vi "Operator Panel 2D_v2.vi"() -> ()   [LabVIEW 2009]
doc: "This VI is an example operator panel.\n\nThe VI contains a table for the field values that may be configured manually, or loaded by checking the \"Prompt for File\" box. The data file should contain 3 columns of data, with each column delimited by a tab character.\n\nBefore the VI is executed, set the desired field units and coordinate system. Once the VI is started, follow the directions in the STATUS indicator to operate. Once a field value is achieved, it will be held indefinitely with no user intervention.\n\nThe present field is displayed in the selected units and coordinate system. The present field is queried once per second.\n\nIf a field point is specified that is outside the limits for the magnet, the VI will abort execution."
uses:
  <vilib>/Utility/file.llb/Read From Spreadsheet File (DBL).vi
panel:
  in  "Z-Axis Communications Config":T1={"GPIB address"=22, "GPIB bus"=1, "connection ID"=refnum, "IP"="192.168.20.40", "Active Comm Interface"=0, "Serial Port"="", "Programmer Type"=0} {"Programmer Type" items=["Model 430", "Model 420"]; "Active Comm Interface" items=["TCP/IP (Model 430 Only)", "RS232", "IEEE488"]}
  in  "Max Ramp Rate - Y Axis (A/s)":dbl=0.065 format="%.3f"
  in  "Max Ramp Rate - Z Axis (A/s)":dbl=0.203 format="%.3f"
  in  "Magnitude Limit (kG)":dbl=45.1 format="%.3f"
  in  "Y-Axis Communications Config":T1={"GPIB address"=22, "GPIB bus"=1, "connection ID"=refnum, "IP"="192.168.20.32", "Active Comm Interface"=0, "Serial Port"="", "Programmer Type"=0} {"Programmer Type" items=["Model 430", "Model 420"]; "Active Comm Interface" items=["TCP/IP (Model 430 Only)", "RS232", "IEEE488"]}
  out "Cartesian Display (T)":T2 {"Z-Axis Field (T)" format="%.3f"; "Y-Axis Field (T)" format="%.3f"}
  in  "Starting index":i32 min=0 max=17 step=1
  in  "Normal color":u32(colorbox)=11711154
  in  "Highlight color":u32(colorbox)=16711680
  out "?":string="American Magnetics, Inc."
  in  "Prompt for File?":bool
  out "Continue Execution?":bool=TRUE
  out "error out":T3
  in  "error in":T3
  out "STATUS":string
  in  "Ramping Control":u16(ring)=3 items=["NEXT VECTOR", "RAMPING", "HOLDING", "PAUSE", "ZERO"]
  out "Cartesian Display (kG)":T4 {"Z-Axis Field (kG)" format="%.3f"; "Y-Axis Field (kG)" format="%.3f"}
  in  "Field Values":string[][](table)
  out "Switch Heaters":bool
  out "Polar Display (T)":T5 {"Z-Axis Field (T)" format="%.3f"; "q (degrees)" format="%.3f"}
  out "Polar Display (kG)":T6 {"Z-Axis Field (kG)" format="%.3f"; "q (degrees)" format="%.3f"}
  in  "Coordinate System":u16(ring) items=["Cartesian", "Polar"]
  in  "Magnetic Field Units":u16(ring) items=["kG", "Tesla"]
  # "Configuration and Status"
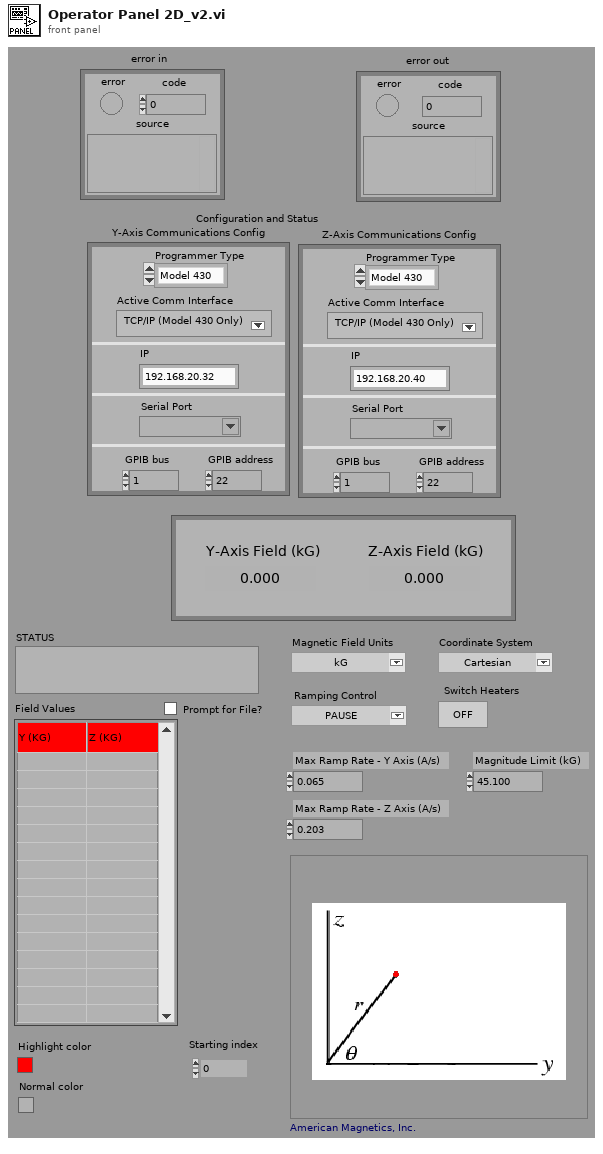
[diagram p1: front panel]
types:
  T1 = cluster{"GPIB address":i16, "GPIB bus":i16, "connection ID":refnum<k5>, "IP":string, "Active Comm Interface":u16, "Serial Port":refnum<visa-resource-name>, "Programmer Type":u16}
  T2 = cluster{"Y-Axis Field (T)":dbl, "Z-Axis Field (T)":dbl}
  T3 = cluster{"error":bool, "code":i32, "source":string}
  T4 = cluster{"Y-Axis Field (kG)":dbl, "Z-Axis Field (kG)":dbl}
  T5 = cluster{"q (degrees)":dbl, "Z-Axis Field (T)":dbl}
  T6 = cluster{"q (degrees)":dbl, "Z-Axis Field (kG)":dbl}
  T7 = enum16{"", "RAMPING", "HOLDING", "PAUSED", "MANUAL UP", "MANUAL DOWN", "ZEROING CURRENT", "QUENCH DETECTED", "HEATING SWITCH"}
  T8 = enum16{"", "RAMPING", "HOLDING", "PAUSED", "MANUAL UP", "MANUAL DOWN", "ZEROING CURRENT", "QUENCH DETECTED", "HEATING SWITCH", "AT ZER0", "COOLING SWITCH"}
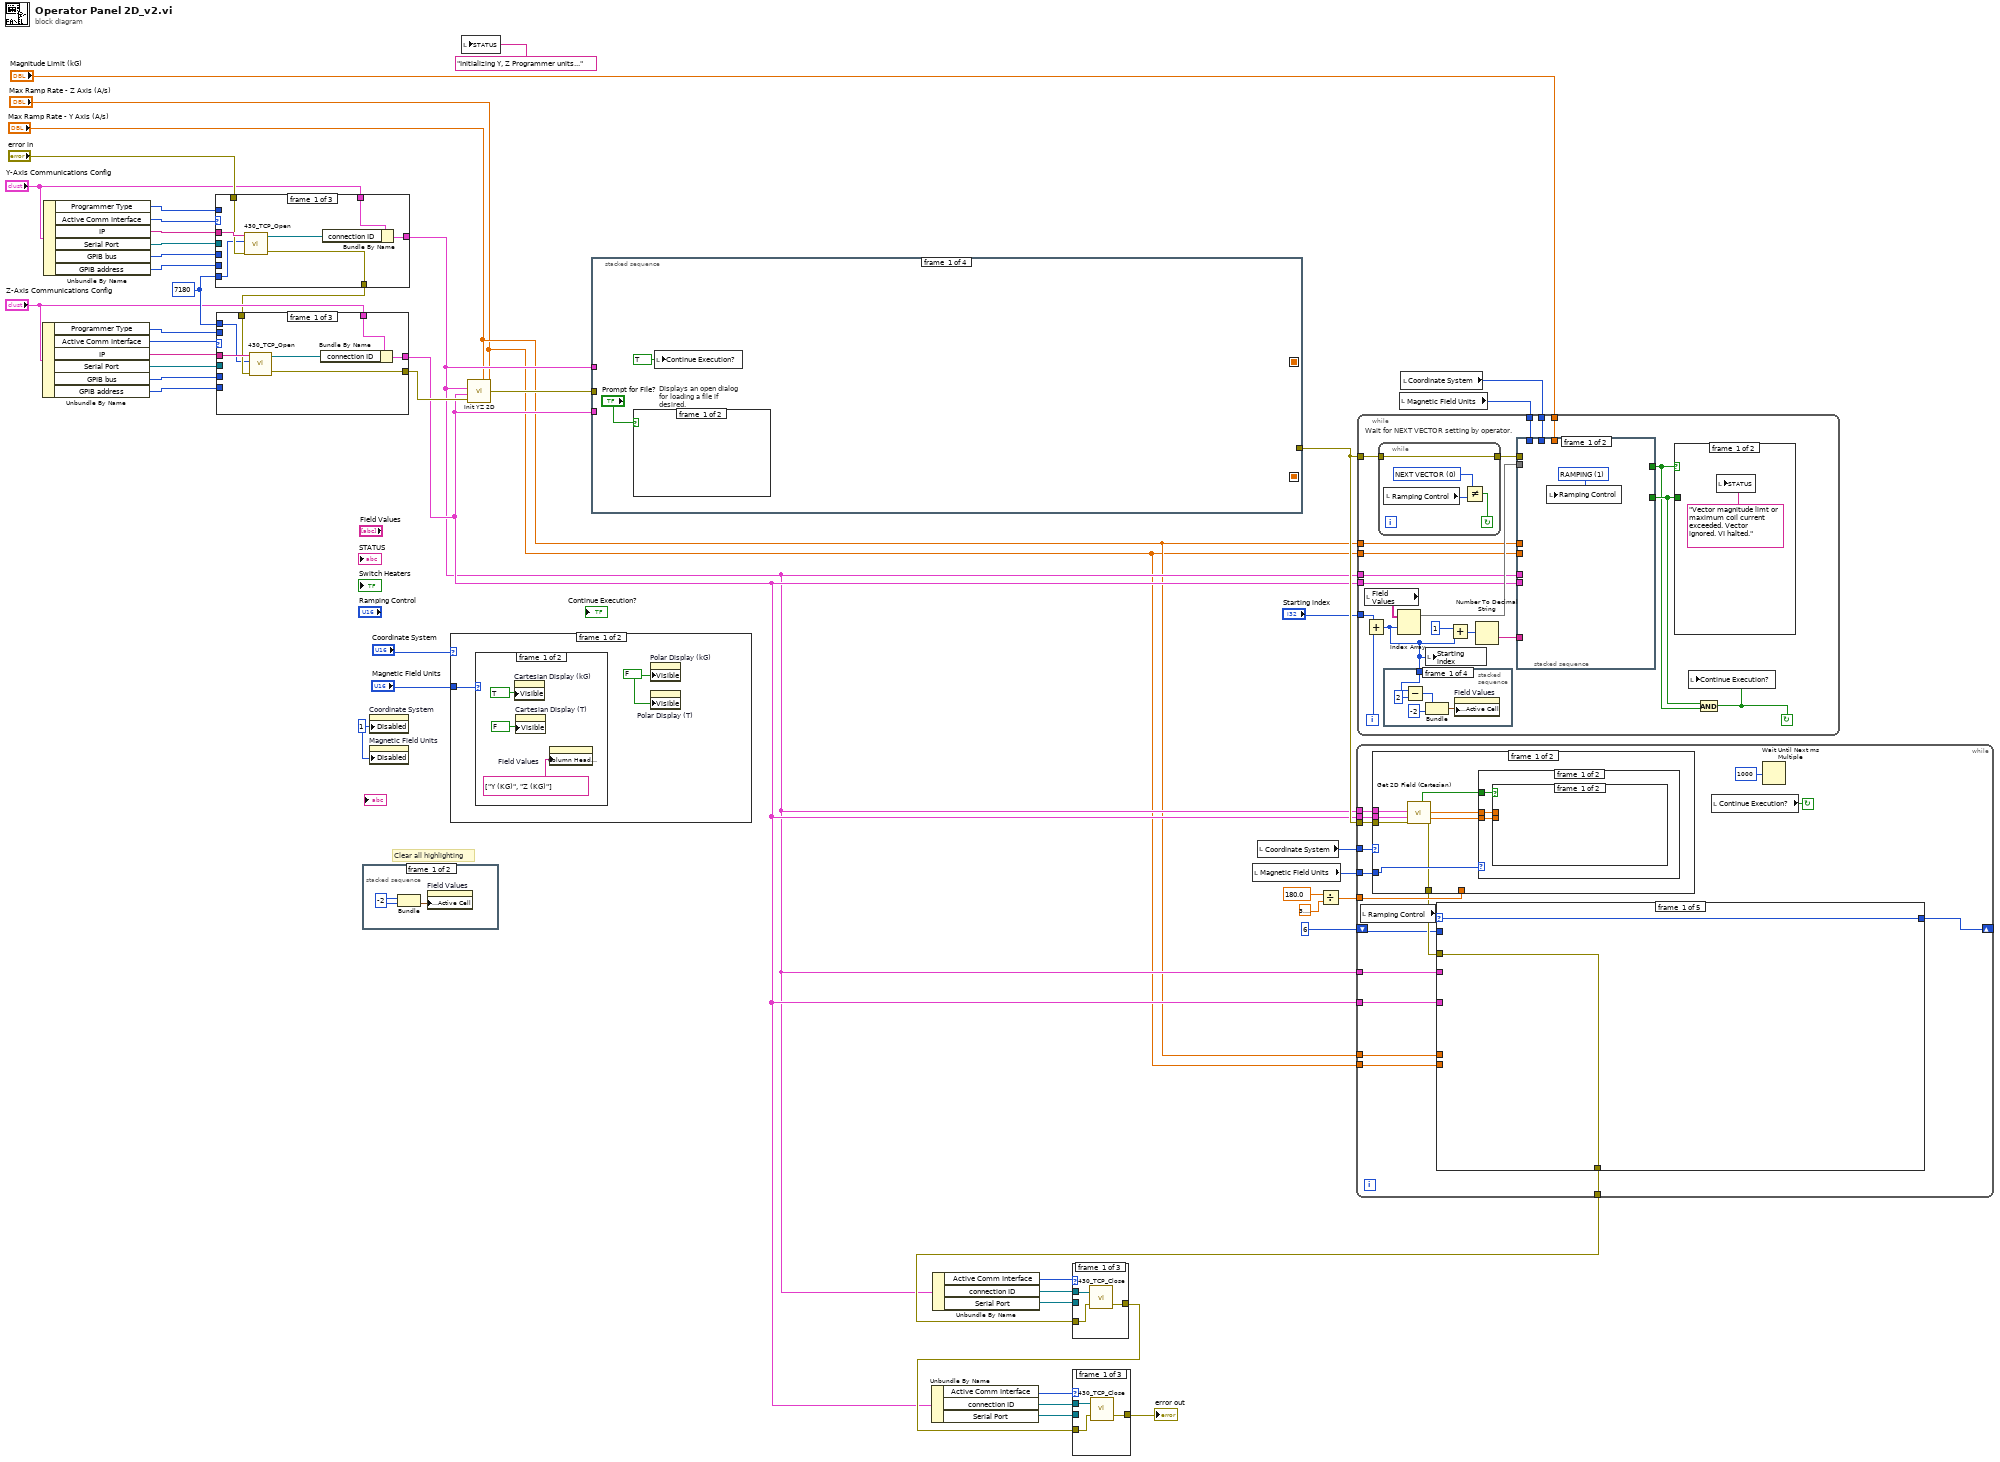
[diagram p0: block diagram]
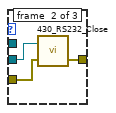
[diagram p2: hidden frame]
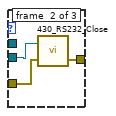
[diagram p4: hidden frame]
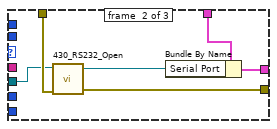
[diagram p6: hidden frame]
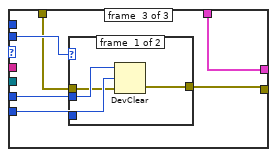
[diagram p7: hidden frame]
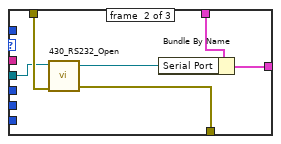
[diagram p9: hidden frame]
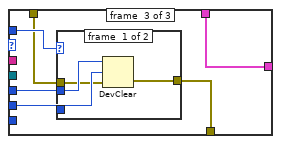
[diagram p10: hidden frame]
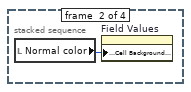
[diagram p12: hidden frame]
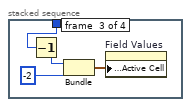
[diagram p13: hidden frame]
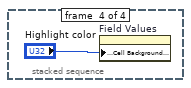
[diagram p14: hidden frame]
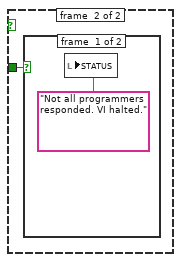
[diagram p15: hidden frame]
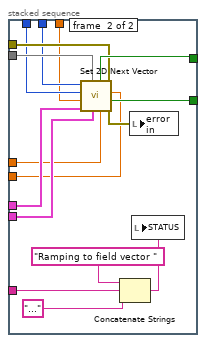
[diagram p17: hidden frame]
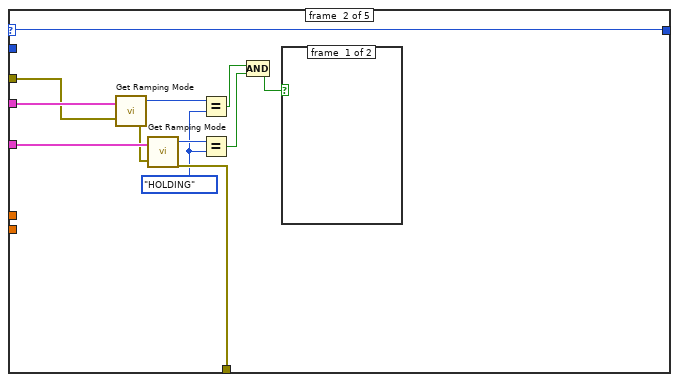
[diagram p18: hidden frame]
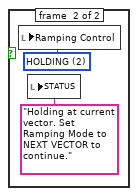
[diagram p19: hidden frame]
diagram:
  w32 = 7180 ("TCP Port")
  w45 = u8 1 ("Write Attribute")
  # "Clear all highlighting"
  n1 = Unbundle By Name("Z-Axis Communications Config") -> ("Programmer Type"=w7:u16, "Active Comm Interface"=w31:u16, "IP"=w28:string, "Serial Port"=w27:refnum<visa-resource-name>, "GPIB bus"=w6:i16, "GPIB address"=w5:i16)
  n2 = Unbundle By Name("Y-Axis Communications Config") -> ("Programmer Type"=w1:u16, "Active Comm Interface"=w30:u16, "IP"=w29:string, "Serial Port"=w26:refnum<visa-resource-name>, "GPIB bus"=w2:i16, "GPIB address"=w3:i16)
  n3 = case shown="2" w30 {
    tunnel: w29 -> [w54 _ _]
    tunnel: "error in" -> [w53 w60 w62]
    tunnel: "Y-Axis Communications Config" -> [w52 w55 w66]
    tunnel: [w50 w58 w66] -> w14
    tunnel: [w49 w59 w61] -> w4
    tunnel: w32 -> [w48 _ _]
    tunnel: w26 -> [_ w56 _]
    tunnel: w3 -> [_ _ w65]
    tunnel: w2 -> [_ _ w64]
    tunnel: w1 -> [_ _ w63]
    frame #0 {
      n4 = call <userlib>:"430_TCP_Open.vi"("IP Address"=w54, "TCP Port"=w48, "error in (no error)"=w53) -> ("connection ID"=w51:refnum<k5>, "error out"=w49:errorcluster)  [unwired: 3 in, 1 out]
      n5 = Bundle By Name(cluster=w52, "connection ID"=w51) -> (w50:T1)
    }
    frame #1 {
      n6 = call <userlib>:"430_RS232_Open.vi"("VISA resource name"=w56, "error in (no error)"=w60) -> ("VISA resource name out"=w57:refnum<visa-resource-name>, "error out"=w59:errorcluster)  [unwired: 5 in]
      n7 = Bundle By Name(cluster=w55, "Serial Port"=w57) -> (w58:T1)
    }
    frame #2 {
      n8 = case shown="0, Default" w63 {
        tunnel: w64 -> [w70 _]
        tunnel: w65 -> [w69 _]
        tunnel: w62 -> [w68 w71]
        tunnel: [w67 w71] -> w61
        frame #0 {
          n9 = DevClear(2:w68, 3:w69, 4:w70) -> (0:w67:errorcluster)  [unwired: 1 out]
        }
        frame #1 {
        }
      }
    }
  }
  n10 = case shown="2" w31 {
    tunnel: w28 -> [w78 _ _]
    tunnel: w4 -> [w77 w84 w86]
    tunnel: [w76 w83 w85] -> w24
    tunnel: "Z-Axis Communications Config" -> [w75 w81 w90]
    tunnel: [w73 w82 w90] -> w15
    tunnel: w32 -> [w72 _ _]
    tunnel: w27 -> [_ w79 _]
    tunnel: w7 -> [_ _ w89]
    tunnel: w6 -> [_ _ w88]
    tunnel: w5 -> [_ _ w87]
    frame #0 {
      n11 = call <userlib>:"430_TCP_Open.vi"("IP Address"=w78, "TCP Port"=w72, "error in (no error)"=w77) -> ("connection ID"=w74:refnum<k5>, "error out"=w76:errorcluster)  [unwired: 3 in, 1 out]
      n12 = Bundle By Name(cluster=w75, "connection ID"=w74) -> (w73:T1)
    }
    frame #1 {
      n13 = call <userlib>:"430_RS232_Open.vi"("VISA resource name"=w79, "error in (no error)"=w84) -> ("VISA resource name out"=w80:refnum<visa-resource-name>, "error out"=w83:errorcluster)  [unwired: 5 in]
      n14 = Bundle By Name(cluster=w81, "Serial Port"=w80) -> (w82:T1)
    }
    frame #2 {
      n15 = case shown="0, Default" w89 {
        tunnel: w88 -> [w94 _]
        tunnel: w87 -> [w93 _]
        tunnel: w86 -> [w92 w95]
        tunnel: [w91 w95] -> w85
        frame #0 {
          n16 = DevClear(2:w92, 3:w93, 4:w94) -> (0:w91:errorcluster)  [unwired: 1 out]
        }
        frame #1 {
        }
      }
    }
  }
  n17 = stacked-sequence {
    frame #0 {
      w96 = -2
      n18 = Bundle(w96, w96) -> (w97:cluster{i32, i32})  [unwired: 1 in]
      n19 = property on="Field Values" class="Tbl (strict)"("Active Cell:Active Cell"=w97) -> ()  [unwired: 2 in, 2 out]
    }
    frame #1 {
      n20 = property on="Field Values" class="Tbl (strict)"("Active Cell:Cell Background Color"="Normal color") -> ()  [unwired: 2 in, 2 out]
    }
  }
  n21 = property on="Coordinate System" class="Ring (strict)"("Disabled"=w45) -> ()  [unwired: 2 in, 2 out]
  n22 = property on="Magnetic Field Units" class="Ring (strict)"("Disabled"=w45) -> ()  [unwired: 2 in, 2 out]
  n23 = case shown="0, Default" "Coordinate System" {
    tunnel: "Magnetic Field Units" -> [w100 w108]
    frame #0 {
      w99 = FALSE ("Write Attribute")
      (unwired) FALSE ("Write Attribute")
      (unwired) TRUE ("Write Attribute")
      n24 = case shown="1" w100 {
        frame #0 {
          n25 = property on="Cartesian Display (kG)" class="Cluster (strict)"("Visible"=TRUE ("Write Attribute")) -> ()  [unwired: 2 in, 2 out]
          n26 = property on="Cartesian Display (T)" class="Cluster (strict)"("Visible"=FALSE ("Write Attribute")) -> ()  [unwired: 2 in, 2 out]
          n27 = property on="Field Values" class="Tbl (strict)"("Column Header Strings[]"=string[] ["Y (KG)", "Z (KG)"] ("Write Attribute")) -> ()  [unwired: 2 in, 2 out]
        }
        frame #1 {
          n28 = property on="Cartesian Display (kG)" class="Cluster (strict)"("Visible"=FALSE ("Write Attribute")) -> ()  [unwired: 2 in, 2 out]
          n29 = property on="Cartesian Display (T)" class="Cluster (strict)"("Visible"=TRUE ("Write Attribute")) -> ()  [unwired: 2 in, 2 out]
          n30 = property on="Field Values" class="Tbl (strict)"("Column Header Strings[]"=string[] ["Y (T)", "Z (T)"] ("Write Attribute")) -> ()  [unwired: 2 in, 2 out]
        }
      }
      n31 = property on="Polar Display (kG)" class="Cluster (strict)"("Visible"=w99) -> ()  [unwired: 2 in, 2 out]
      n32 = property on="Polar Display (T)" class="Cluster (strict)"("Visible"=w99) -> ()  [unwired: 2 in, 2 out]
    }
    frame #1 {
      (unwired) FALSE ("Write Attribute")
      (unwired) TRUE ("Write Attribute")
      w107 = FALSE ("Write Attribute")
      n33 = case shown="0, Default" w108 {
        frame #0 {
          n34 = property on="Polar Display (kG)" class="Cluster (strict)"("Visible"=TRUE ("Write Attribute")) -> ()  [unwired: 2 in, 2 out]
          n35 = property on="Polar Display (T)" class="Cluster (strict)"("Visible"=FALSE ("Write Attribute")) -> ()  [unwired: 2 in, 2 out]
          n36 = property on="Field Values" class="Tbl (strict)"("Column Header Strings[]"=string[] ["Mag. r (KG)", "Theta (deg)"] ("Write Attribute")) -> ()  [unwired: 2 in, 2 out]
        }
        frame #1 {
          n37 = property on="Polar Display (kG)" class="Cluster (strict)"("Visible"=FALSE ("Write Attribute")) -> ()  [unwired: 2 in, 2 out]
          n38 = property on="Polar Display (T)" class="Cluster (strict)"("Visible"=TRUE ("Write Attribute")) -> ()  [unwired: 2 in, 2 out]
          n39 = property on="Field Values" class="Tbl (strict)"("Column Header Strings[]"=string[] ["Mag. r (T)", "Theta (deg)"] ("Write Attribute")) -> ()  [unwired: 2 in, 2 out]
        }
      }
      n40 = property on="Cartesian Display (kG)" class="Cluster (strict)"("Visible"=w107) -> ()  [unwired: 2 in, 2 out]
      n41 = property on="Cartesian Display (T)" class="Cluster (strict)"("Visible"=w107) -> ()  [unwired: 2 in, 2 out]
    }
  }
  n42 = local write "STATUS"("Initializing Y, Z Programmer units..." ("STATUS")) -> ()
  n43 = call <userlib>:"Init YZ 2D.vi"("Max Ramp Rate Z-axis"="Max Ramp Rate - Z Axis (A/s)", "Max Ramp Rate Y-axis"="Max Ramp Rate - Y Axis (A/s)", "error in"=w24, "Z-Axis Communications Config"=w15, "Y-Axis Communications Config"=w14) -> ("error out"=w43:T3)  [unwired: 5 in]
  n44 = stacked-sequence {
    seq-local: [_ w122 _ _] -> [_ _ w169 _]
    seq-local: [_ w121 _ _] -> [_ _ w168 _]
    tunnel: w15 -> [_ w124 _ _]
    tunnel: w43 -> [_ w125 _ _]
    tunnel: [_ w120 _ _] -> w39
    tunnel: w14 -> [_ w123 _ _]
    frame #0 {
      n45 = case "Displays an open dialog for loading a file if desired." shown="True" "Prompt for File?" {
        frame #0 {
        }
        frame #1 {
          n46 = call-poly <vilib>:"Read From Spreadsheet File.vi"() -> ("all rows"=w119:dbl[][])  [unwired: 7 in, 4 out]
          n47 = Number To Fractional String(number=w119, precision (6)=i16 4) -> (F-format string=w118:string[][])  [unwired: 2 in]
          n48 = local write "Field Values"(w118) -> ()
        }
      }
      n49 = local write "Continue Execution?"(TRUE ("Continue Execution?")) -> ()
    }
    frame #1 {
      w133 = u16 3 items=["NEXT VECTOR", "RAMPING", "HOLDING", "PAUSE", "ZERO"] ("Ramping Control")
      n50 = call <userlib>:"Get Switch Present.vi"("error in"=w125, "Communications Config"=w123) -> ("error out"=w129:T3, "Switch Present?"=w130:bool)
      n51 = case shown="True" w130 {
        tunnel: w129 -> [w151 w160]
        tunnel: w123 -> [_ w153]
        tunnel: [0.0 w157] -> w121
        tunnel: [w151 w159] -> w128
        frame #0 {
        }
        frame #1 {
          n52 = call <userlib>:"Get Switch Heater Time.vi"("error in"=w160, "Communications Config"=w153) -> ("error out"=w156:T3, "Switch Heating Time (secs)"=w158:dbl)
          n53 = call <userlib>:"Get Switch Heater.vi"("error in"=w156, "Communications Config"=w153) -> ("error out"=w155:T3, "Switch Heater Indicator"=w154:bool)
          n54 = case shown="False" w154 {
            tunnel: [w165 w166] -> w159
            tunnel: w158 -> [w163 _]
            tunnel: [w163 0.0] -> w157
            tunnel: w155 -> [w161 w166]
            tunnel: w153 -> [w162 _]
            frame #0 {
              n55 = call <userlib>:"Set Switch Heater.vi"("error in"=w161, "Switch Heater Control"=TRUE, "Communications Config"=w162) -> ("error out"=w165:T3)
            }
            frame #1 {
            }
          }
        }
      }
      n56 = call <userlib>:"Get Switch Present.vi"("error in"=w128, "Communications Config"=w124) -> ("error out"=w126:T3, "Switch Present?"=w127:bool)
      n57 = case shown="True" w127 {
        tunnel: w126 -> [w134 w143]
        tunnel: w124 -> [_ w136]
        tunnel: [0.0 w140] -> w122
        tunnel: [w134 w142] -> w120
        frame #0 {
        }
        frame #1 {
          n58 = call <userlib>:"Get Switch Heater Time.vi"("error in"=w143, "Communications Config"=w136) -> ("error out"=w139:T3, "Switch Heating Time (secs)"=w141:dbl)
          n59 = call <userlib>:"Get Switch Heater.vi"("error in"=w139, "Communications Config"=w136) -> ("error out"=w138:T3, "Switch Heater Indicator"=w137:bool)
          n60 = case shown="False" w137 {
            tunnel: [w144 w149] -> w142
            tunnel: w141 -> [w147 _]
            tunnel: [w147 0.0] -> w140
            tunnel: w138 -> [w145 w149]
            tunnel: w136 -> [w146 _]
            frame #0 {
              n61 = call <userlib>:"Set Switch Heater.vi"("error in"=w145, "Switch Heater Control"=TRUE, "Communications Config"=w146) -> ("error out"=w144:T3)
            }
            frame #1 {
            }
          }
        }
      }
      n62 = local write "Ramping Control"(w133) -> ()
      n63 = local write "Switch Heaters"(TRUE ("Switch Heater Control")) -> ()
      n64 = property on="Switch Heaters" class="Boolean (strict)"("Disabled"=u8 1 ("Write Attribute")) -> ()  [unwired: 2 in, 2 out]
    }
    frame #2 {
      n65 = Max & Min(x=w169, y=w168) -> (max(x,y)=w170:dbl)  [unwired: 1 out]
      n66 = local write "STATUS"("Heating switches..." ("STATUS")) -> ()
      n67 = Add(x=w170, y=2) -> (x+y=w174:dbl)
      n68 = property on="Ramping Control" class="Ring (strict)"("Disabled"=u8 1 ("Write Attribute")) -> ()  [unwired: 2 in, 2 out]
      n69 = Multiply(x=w174, y=1000) -> (x*y=w173:dbl)
      n70 = Wait (ms)(milliseconds to wait=w173) -> ()  [unwired: 1 out]
    }
    frame #3 {
      n71 = property on="Ramping Control" class="Ring (strict)"("Disabled"=u8 0 ("Write Attribute")) -> ()  [unwired: 2 in, 2 out]
      n72 = local write "STATUS"("Ready to ramp to first vector. Set Ramping Mode to NEXT VECTOR to begin." ("STATUS")) -> ()
    }
  }
  n73 = Unbundle By Name(w15) -> ("Active Comm Interface"=w21:u16, "connection ID"=w20:refnum<k5>, "Serial Port"=w19:refnum<visa-resource-name>)
  n74 = Unbundle By Name(w14) -> ("Active Comm Interface"=w22:u16, "connection ID"=w18:refnum<k5>, "Serial Port"=w17:refnum<visa-resource-name>)
  n75 = local read "Magnetic Field Units"() -> (w38:u16)
  n76 = local read "Coordinate System"() -> (w40:u16)
  n77 = Divide(x=180.0, y=3.141592653589793) -> (x/y=w35:dbl)
  n78 = while {
    shift-left: u16 6 ("Ramping Control") -> [w181]
    shift-right: [w182] -> _
    tunnel: [w184] -> w16
    tunnel: w15 -> [w186]
    tunnel: w14 -> [w187]
    tunnel: w35 -> [w189]
    tunnel: w38 -> [w190]
    tunnel: w39 -> [w191]
    tunnel: w15 -> [w192]
    tunnel: w14 -> [w193]
    tunnel: w40 -> [w194]
    tunnel: "Max Ramp Rate - Y Axis (A/s)" -> [w180]
    tunnel: "Max Ramp Rate - Z Axis (A/s)" -> [w179]
    stop <- w183 continue-if-true
    n79 = local read "Ramping Control"() -> (w188:u16)
    n80 = case shown="0, Default" w194 {
      tunnel: w193 -> [w257 w281]
      tunnel: w192 -> [w256 w280]
      tunnel: w191 -> [w255 w279]
      tunnel: w190 -> [w254 w278]
      tunnel: w189 -> [_ w275]
      tunnel: [w250 w273] -> w185
      frame #0 {
        n81 = call <userlib>:"Get 2D Field (Cartesian).vi"("Y-Axis Communications Config"=w257, "Z-Axis Communications Config"=w256, "error in"=w255) -> ("All Instruments Responded?"=w251:bool, "Y-Axis Field (kG)"=w253:dbl, "Z-Axis Field (kG)"=w252:dbl, "error out"=w250:T3)  [unwired: 2 in]
        n82 = case shown="0, Default" w254 {
          tunnel: w253 -> [w260 w266]
          tunnel: w252 -> [w259 w267]
          tunnel: w251 -> [w258 w269]
          frame #0 {
            n83 = case shown="True" w258 {
              tunnel: w260 -> [_ w262]
              tunnel: w259 -> [_ w261]
              frame #0 {
              }
              frame #1 {
                n84 = Bundle("Y-Axis Field (kG)"=w262, "Z-Axis Field (kG)"=w261) -> (→"Cartesian Display (kG)":T4)  [unwired: 1 in]
              }
            }
          }
          frame #1 {
            w268 = 0.1 ("y")
            n85 = Multiply(x=w266, y=w268) -> (x*y=w265:dbl)
            n86 = Multiply(x=w267, y=w268) -> (x*y=w264:dbl)
            n87 = case shown="True" w269 {
              tunnel: w265 -> [_ w272]
              tunnel: w264 -> [_ w271]
              frame #0 {
              }
              frame #1 {
                n88 = Bundle(w272, w271) -> (→"Cartesian Display (T)":cluster{dbl, dbl})  [unwired: 1 in]
              }
            }
          }
        }
      }
      frame #1 {
        n89 = call <userlib>:"Get 2D Field (Polar).vi"("Y-Axis Communications Config"=w281, "Z-Axis Communications Config"=w280, "error in"=w279) -> ("All Instruments Responded?"=w274:bool, "Radial (r) Field (kG)"=w277:dbl, "q (radians)"=w276:dbl, "error out"=w273:T3)  [unwired: 2 in]
        n90 = case shown="0, Default" w278 {
          tunnel: w277 -> [w286 w295]
          tunnel: w276 -> [w284 w294]
          tunnel: w275 -> [w283 w293]
          tunnel: w274 -> [w285 w292]
          frame #0 {
            n91 = Multiply(x=w284, y=w283) -> (x*y=w282:dbl)
            n92 = case shown="True" w285 {
              tunnel: w286 -> [_ w289]
              tunnel: w282 -> [_ w288]
              frame #0 {
              }
              frame #1 {
                n93 = Bundle("Radial (r) Field (kG)"=w289, w288) -> (→"Polar Display (kG)":cluster{"Radial (r) Field (kG)":dbl, dbl})  [unwired: 1 in]
              }
            }
          }
          frame #1 {
            n94 = Multiply(x=w295, y=0.1) -> (x*y=w291:dbl)
            n95 = Multiply(x=w294, y=w293) -> (x*y=w290:dbl)
            n96 = case shown="True" w292 {
              tunnel: w291 -> [_ w299]
              tunnel: w290 -> [_ w298]
              frame #0 {
              }
              frame #1 {
                n97 = Bundle(w299, w298) -> (→"Polar Display (T)":cluster{dbl, dbl})  [unwired: 1 in]
              }
            }
          }
        }
      }
    }
    n98 = case shown="3" w188 {
      selector: w188 -> [w196 w206 w213 w216 w231]
      tunnel: w187 -> [_ w209 _ w220 w237]
      tunnel: w186 -> [_ w208 _ w219 w236]
      tunnel: w185 -> [w197 w201 w212 w218 w235]
      tunnel: [w197 w207 w212 w217 w234] -> w184
      tunnel: [w196 w206 w213 w216 w231] -> w182
      tunnel: w181 -> [_ _ _ w215 w233]
      tunnel: w180 -> [_ _ _ _ w230]
      tunnel: w179 -> [_ _ _ _ w229]
      frame #0 {
      }
      frame #1 {
        w200 = T7."HOLDING" ("y")
        n99 = call <userlib>:"Get Ramping Mode.vi"("Communications Config"=w209, "error in"=w201) -> ("Ramping Mode"=w204:T8, "error out"=w205:T3)  [unwired: 1 out]
        n100 = call <userlib>:"Get Ramping Mode.vi"("Communications Config"=w208, "error in"=w205) -> ("Ramping Mode"=w203:T8, "error out"=w207:T3)  [unwired: 1 out]
        n101 = Equal?(x=w204, y=w200) -> (x = y?=w199:bool)
        n102 = Equal?(x=w203, y=w200) -> (x = y?=w198:bool)
        n103 = Compound Arithmetic op=AND(w199, w198) -> (w202:bool)
        n104 = case shown="True" w202 {
          frame #0 {
          }
          frame #1 {
            w211 = u16 2 items=["NEXT VECTOR", "RAMPING", "HOLDING", "PAUSE", "ZERO"] ("Ramping Control")
            n105 = local write "Ramping Control"(w211) -> ()
            n106 = local write "STATUS"("Holding at current vector. Set Ramping Mode to NEXT VECTOR to continue." ("STATUS")) -> ()
          }
        }
      }
      frame #2 {
      }
      frame #3 {
        n107 = Not Equal?(x=w216, y=w215) -> (x != y?=w214:bool)
        n108 = case shown="True" w214 {
          tunnel: w220 -> [_ w228]
          tunnel: w219 -> [_ w227]
          tunnel: w218 -> [w221 w222]
          tunnel: [w221 w225] -> w217
          frame #0 {
          }
          frame #1 {
            w223 = u16 1 items=["RAMP", "PAUSE", "MANUAL UP", "MANUAL DOWN", "ZERO"] ("Ramping Mode")
            n109 = call <userlib>:"Set Ramping Mode.vi"("error in"=w222, "Ramping Mode"=w223, "Communications Config"=w228) -> ("error out"=w226:T3)
            n110 = call <userlib>:"Set Ramping Mode.vi"("error in"=w226, "Ramping Mode"=w223, "Communications Config"=w227) -> ("error out"=w225:T3)
            n111 = local write "STATUS"("All Programmers are PAUSED. Set Ramping Mode to NEXT VECTOR to continue." ("STATUS")) -> ()
          }
        }
      }
      frame #4 {
        n112 = Not Equal?(x=w231, y=w233) -> (x != y?=w232:bool)
        n113 = case shown="True" w232 {
          tunnel: w237 -> [_ w245]
          tunnel: w236 -> [_ w244]
          tunnel: w235 -> [w238 w247]
          tunnel: [w238 w240] -> w234
          tunnel: w230 -> [_ w243]
          tunnel: w229 -> [_ w242]
          frame #0 {
          }
          frame #1 {
            w239 = u16 4 items=["RAMP", "PAUSE", "MANUAL UP", "MANUAL DOWN", "ZERO"] ("Ramping Mode")
            n114 = local write "STATUS"("Zeroing vector." ("STATUS")) -> ()
            n115 = call <userlib>:"Set Ramping Mode.vi"("error in"=w247, "Ramping Mode"=w239, "Communications Config"=w245) -> ("error out"=w249:T3)
            n116 = call <userlib>:"Set Ramping Mode.vi"("error in"=w249, "Ramping Mode"=w239, "Communications Config"=w244) -> ("error out"=w241:T3)
            n117 = call <userlib>:"Set Current Ramp Rate.vi"("Communications Config"=w245, "Ramp Rate (A/sec)"=w243, "error in"=w241) -> ("error out"=w246:T3)  [unwired: 2 in]
            n118 = call <userlib>:"Set Current Ramp Rate.vi"("Communications Config"=w244, "Ramp Rate (A/sec)"=w242, "error in"=w246) -> ("error out"=w240:T3)  [unwired: 2 in]
          }
        }
      }
    }
    n119 = local read "Continue Execution?"() -> (w183:bool)
    n120 = Wait Until Next ms Multiple(millisecond multiple=u32 1000) -> ()  [unwired: 1 out]
  }
  n121 = case shown="0, Default" w22 {
    tunnel: w18 -> [w302 _ _]
    tunnel: w16 -> [w301 w305 w306]
    tunnel: [w300 w304 w306] -> w23
    tunnel: w17 -> [_ w303 _]
    frame #0 {
      n122 = call <userlib>:"430_TCP_Close.vi"("error in (no error)"=w301, "connection ID"=w302) -> ("error out"=w300:errorcluster)  [unwired: 1 out]
    }
    frame #1 {
      n123 = call <userlib>:"430_RS232_Close.vi"("error in (no error)"=w305, "VISA resource name"=w303) -> ("error out"=w304:errorcluster)  [unwired: 1 in]
    }
    frame #2 {
    }
  }
  n124 = case shown="0, Default" w21 {
    tunnel: w20 -> [w309 _ _]
    tunnel: w23 -> [w308 w312 w313]
    tunnel: [w307 w311 w313] -> w13
    tunnel: w19 -> [_ w310 _]
    frame #0 {
      n125 = call <userlib>:"430_TCP_Close.vi"("error in (no error)"=w308, "connection ID"=w309) -> ("error out"=w307:errorcluster)  [unwired: 1 out]
    }
    frame #1 {
      n126 = call <userlib>:"430_RS232_Close.vi"("error in (no error)"=w312, "VISA resource name"=w310) -> ("error out"=w311:errorcluster)  [unwired: 1 in]
    }
    frame #2 {
    }
  }
  "error out" <- w13
  n127 = local read "Magnetic Field Units"() -> (w41:u16)
  n128 = local read "Coordinate System"() -> (w42:u16)
  n129 = while {
    tunnel: "Starting index" -> [w319]
    tunnel: w15 -> [w325]
    tunnel: w14 -> [w326]
    tunnel: w41 -> [w327]
    tunnel: w42 -> [w328]
    tunnel: w39 -> [w331]
    tunnel: "Max Ramp Rate - Y Axis (A/s)" -> [w315]
    tunnel: "Max Ramp Rate - Z Axis (A/s)" -> [w314]
    tunnel: "Magnitude Limit (kG)" -> [w316]
    i -> [w318]
    stop <- w320 continue-if-true
    n130 = local read "Field Values"() -> (w322:string[][])
    n131 = Add(x=w319, y=w318) -> (x+y=w317:i32)
    n132 = while "Wait for NEXT VECTOR setting by operator." {
      tunnel: [w335] -> w330
      tunnel: w331 -> [w335]
      stop <- w336 continue-if-true
      w334 = u16 0 items=["NEXT VECTOR", "RAMPING", "HOLDING", "PAUSE", "ZERO"] ("Ramping Control")
      n133 = local read "Ramping Control"() -> (w337:u16)
      n134 = Not Equal?(x=w334, y=w337) -> (x != y?=w336:bool)
    }
    n135 = stacked-sequence {
      tunnel: w317 -> [w339 _ w345 _]
      frame #0 {
        (unwired) -2
        n136 = Subtract(x=w339, y=2) -> (x-y=w342:i32)
        n137 = Bundle(w342, -2) -> (w340:cluster{i32, i32})  [unwired: 1 in]
        n138 = property on="Field Values" class="Tbl (strict)"("Active Cell:Active Cell"=w340) -> ()  [unwired: 2 in, 2 out]
      }
      frame #1 {
        n139 = local read "Normal color"() -> (w343:u32)
        n140 = property on="Field Values" class="Tbl (strict)"("Active Cell:Cell Background Color"=w343) -> ()  [unwired: 2 in, 2 out]
      }
      frame #2 {
        n141 = Decrement(x=w345) -> (x-1=w344:i32)
        n142 = Bundle(w344, -2) -> (w347:cluster{i32, i32})  [unwired: 1 in]
        n143 = property on="Field Values" class="Tbl (strict)"("Active Cell:Active Cell"=w347) -> ()  [unwired: 2 in, 2 out]
      }
      frame #3 {
        n144 = property on="Field Values" class="Tbl (strict)"("Active Cell:Cell Background Color"="Highlight color") -> ()  [unwired: 2 in, 2 out]
      }
    }
    n145 = Index Array(array=w322, index (row)=w317) -> (element=w329:string[])  [unwired: 1 in]
    n146 = local write "Starting index"(w317) -> ()
    n147 = Add(x=1, y=w317) -> (x+y=w332:i32)
    n148 = Number To Decimal String(number=w332) -> (decimal integer string=w321:string)  [unwired: 1 in]
    n149 = stacked-sequence {
      tunnel: [_ w368] -> w323
      tunnel: [_ w367] -> w324
      tunnel: w330 -> [_ w363]
      tunnel: w329 -> [_ w362]
      tunnel: w328 -> [_ w361]
      tunnel: w327 -> [_ w360]
      tunnel: w326 -> [_ w359]
      tunnel: w325 -> [_ w358]
      tunnel: w321 -> [_ w357]
      tunnel: w316 -> [_ w355]
      tunnel: w315 -> [_ w354]
      tunnel: w314 -> [_ w353]
      frame #0 {
        w352 = u16 1 items=["NEXT VECTOR", "RAMPING", "HOLDING", "PAUSE", "ZERO"] ("Ramping Control")
        n150 = local write "Ramping Control"(w352) -> ()
      }
      frame #1 {
        n151 = call <userlib>:"Set 2D Next Vector.vi"("Max Ramp Rate - Z Axis (A/s)"=w353, "error in"=w363, "Max Ramp Rate - Y Axis (A/s)"=w354, "Z-Axis Communications Config"=w358, "Input Vector"=w362, "Y-Axis Communications Config"=w359, "Magnitude Limit (kG)"=w355, "Magnetic Field Units"=w360, "Coordinate System"=w361) -> ("error out"=w356:T3, "All Instruments Responded?"=w367:bool, "Within Limits?"=w368:bool)
        n152 = Concatenate Strings("Ramping to field vector " ("STATUS"), w357, "..." ("STATUS")) -> (w364:string)
        n153 = local write "error in"(w356) -> ()
        n154 = local write "STATUS"(w364) -> ()
      }
    }
    n155 = case shown="True" w323 {
      tunnel: w324 -> [_ w350]
      frame #0 {
        n156 = local write "STATUS"("Vector magnitude limt or maximum coil current exceeded. Vector ignored. VI halted." ("STATUS")) -> ()
      }
      frame #1 {
        n157 = case shown="False" w350 {
          frame #0 {
            n158 = local write "STATUS"("Not all programmers responded. VI halted." ("STATUS")) -> ()
          }
          frame #1 {
          }
        }
      }
    }
    n159 = Compound Arithmetic op=AND(w324, w323) -> (w320:bool)
    n160 = local write "Continue Execution?"(w320) -> ()
  }
